vi "1D CrossCorrelation.vi"(1 "Intensity Profile":dbl[](array[numeric]) format="%.2f") -> (0 "CrossCorrelation":dbl[](array[numeric]) format="%.2f")   [LabVIEW 2011, in "OfflineTracker.lvlib"]
uses:
  <vilib>/Analysis/2dsp.llb/Inverse Complex FFT.vi
  <vilib>/Analysis/2dsp.llb/Real FFT.vi
  OfflineTracker.lvlib
  <vilib>/Analysis/NI_AALPro.lvlib
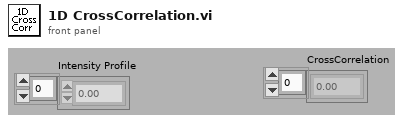
[diagram p1: front panel]
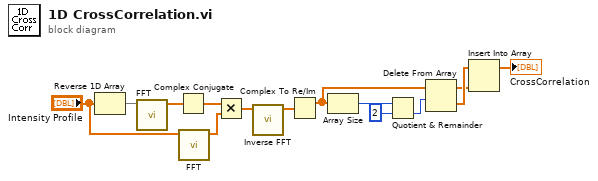
[diagram p0: block diagram]
diagram:
  n1 = Reverse 1D Array(array="Intensity Profile") -> (reversed array=w14:dbl[])
  n2 = call-poly <vilib>:"FFT.vi"("X"=w14) -> ("FFT {X}"=w13:cdb[])  [unwired: 2 in, 8 out]
  n3 = Complex Conjugate(1:w13) -> (0:w9:cdb[])
  n4 = call-poly <vilib>:"FFT.vi"("X"="Intensity Profile") -> ("FFT {X}"=w10:cdb[])  [unwired: 2 in, 8 out]
  n5 = Multiply(x=w9, y=w10) -> (x*y=w12:cdb[])
  n6 = call-poly <vilib>:"Inverse FFT.vi"("FFT {X}"=w12) -> ("X"=w11:cdb[])  [unwired: 1 in, 9 out]
  n7 = Complex To Re/Im(x + iy=w11) -> (x=w4:dbl[])  [unwired: 1 out]
  n8 = Array Size(array=w4) -> (size(s)=w2:i32)
  n9 = Quotient & Remainder(x=w2, y=2) -> (floor(x/y)=w3:i32)  [unwired: 1 out]
  n10 = Delete From Array(array=w4, length=w3) -> (deleted portion=w7:dbl[], array with subset deleted=w6:dbl[])  [unwired: 1 in]
  n11 = Insert Into Array(array=w7, new element=w6) -> (→"CrossCorrelation":dbl[])  [unwired: 1 in]
